vi "Test PGSQL.vi"() -> ()   [LabVIEW 2019, in "Logger.PGSQL.lvclass"]
uses:
  Logger.PGSQL.lvclass
panel:
  in  "stop":bool
  in  "String":string
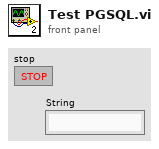
[diagram p1: front panel]
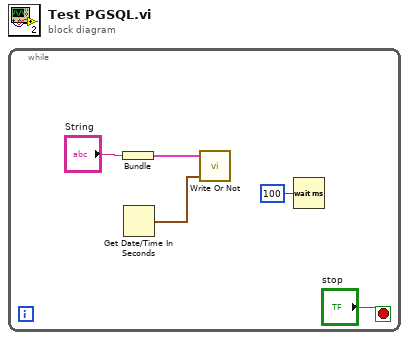
[diagram p0: block diagram]
diagram:
  n1 = while {
    stop <- "stop" stop-if-true
    n2 = Bundle("String"="String") -> (w1:cluster{"String":string})  [unwired: 1 in]
    n3 = Get Date/Time In Seconds() -> (seconds since 1Jan1904=w4:timestamp)
    n4 = call "Write Or Not.vi"("Time"=w4, "data in"=w1) -> ()  [unwired: 1 in, 1 out]
    n5 = Wait (ms)(milliseconds to wait=u32 100) -> ()  [unwired: 1 out]
  }
